vi "img_write_image.vi"(8 "error in":errorcluster, 9 "Sector size (512)":u32=512, 10 "Image In":T1, 11 "hFile":i64) -> (0 "error out":errorcluster, 1 "lpNumberOfBytesWritten":u32, 2 "Image Out":T1, 3 "hFile out":i64)   [LabVIEW 2016]
doc: "This VI writes an image to file using the Win API function WriteFile()."
uses:
  <vilib>/vision/Image Controls.llb/IMAQ Image.ctl
  kernel32.dll
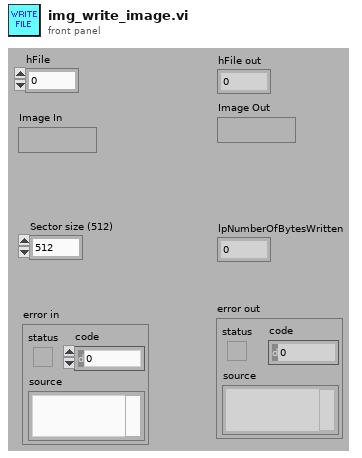
[diagram p1: front panel]
types:
  T1 = typedef "IMAQ Image.ctl" = refnum<image>
  T2 = enum32{"Map Pixel Pointer", "Unmap Pixel Pointer", "Get Pixels Infos"}
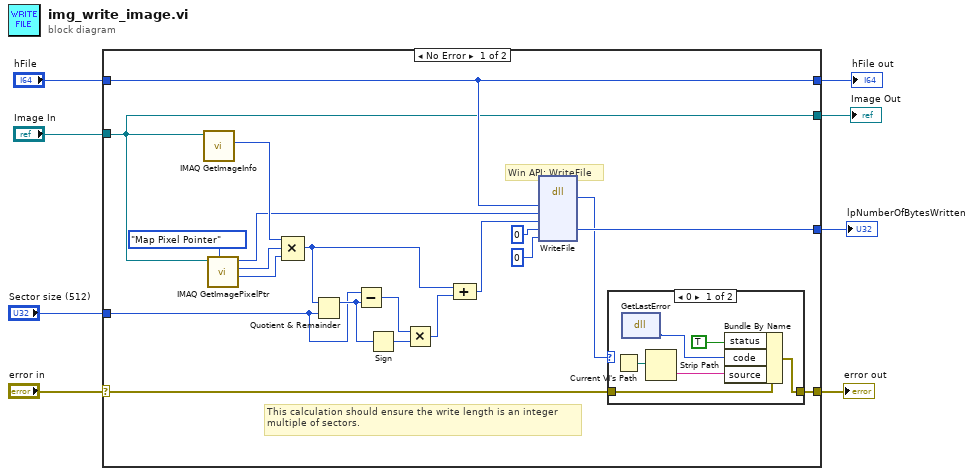
[diagram p0: block diagram]
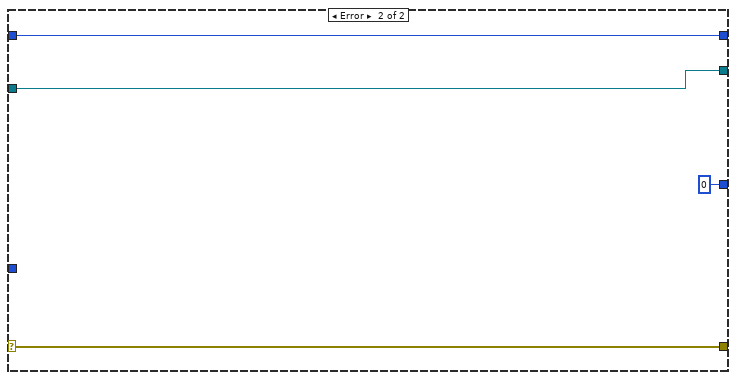
[diagram p3: hidden frame]
diagram:
  n1 = case shown="No Error" "error in" {
    selector: "error in" -> [w14 w38]
    tunnel: "hFile" -> [w12 w37]
    tunnel: "Image In" -> [w11 w36]
    tunnel: [w26 u32 0 ("lpNumberOfBytesWritten")] -> w7
    tunnel: [w25 w38] -> w6
    tunnel: "Sector size (512)" -> [w13 _]
    tunnel: [w12 w37] -> w2
    tunnel: [w11 w36] -> w1
    frame No Error {
      # "This calculation should ensure the write length is an integer\nmultiple of sectors."
      # "Win API: WriteFile"
      n2 = call "IMAQ GetImageInfo"("Image"=w11) -> ("Y Resolution"=w22:i32)  [unwired: 1 in, 9 out]
      n3 = call "IMAQ GetImagePixelPtr"("Function"=T2."Map Pixel Pointer", "Image"=w11) -> ("Pixel Size (Bytes)"=w23:i32, "LineWidth(Pixels)"=w24:i32, "Pixel Pointer out"=w10:u64)  [unwired: 4 in, 3 out]
      n4 = Compound Arithmetic op=MULTIPLY(w22, w24, w23) -> (w21:i32)
      n5 = Quotient & Remainder(x=w21, y=w13) -> (x-y*floor(x/y)=w15:u32)  [unwired: 1 out]
      n6 = Subtract(x=w13, y=w15) -> (x-y=w17:u32)
      n7 = Sign(1:w15) -> (0:w18:u32)
      n8 = Multiply(x=w17, y=w18) -> (x*y=w16:u32)
      n9 = Compound Arithmetic op=ADD(w21, w16) -> (w20:u32)
      n10 = dll-call lib="kernel32.dll" fn="WriteFile"("hFile"=w12, "lpBuffer"=w10, "nNumberOfBytesToWrite"=w20, "lpNumberOfBytesWritten"=u32 0, "lpOverlapped"=u32 0) -> ("error"=w9:i32, "lpNumberOfBytesWritten"=w26:u32)  [unwired: 6 in, 3 out]
      n11 = case shown="0" w9 {
        tunnel: w14 -> [w34 w35]
        tunnel: [w33 w35] -> w25
        frame 0 {
          n12 = Current VI's Path() -> (path=w31:path)
          n13 = dll-call lib="kernel32.dll" fn="GetLastError"() -> ("error"=w29:u32)  [unwired: 3 in, 2 out]
          n14 = Strip Path(path=w31) -> (name=w30:string)  [unwired: 1 out]
          n15 = Bundle By Name(cluster=w34, "status"=TRUE, "code"=w29, "source"=w30) -> (w33:errorcluster)
        }
        frame 1, Default {
        }
      }
    }
    frame Error {
    }
  }
  "Image Out" <- w1
  "lpNumberOfBytesWritten" <- w7
  "hFile out" <- w2
  "error out" <- w6
